vi "RDUW_2.0(old).vi"() -> ()   [LabVIEW 2010]
uses:
  <vilib>/express/express arith-compare/Formula/XNode/ExpressFormulaBlockNode.xnode
panel:
  in  "Current (mA)":dbl
  in  "Laser GPIB":u8=10 max=100
  out "Dummy":string
  out "Dummy angle":i16[](array[numeric])
  out "Quadrant":u8
  out "move y":i32
  out "move x":i32
  out "b":dbl
  out "a":dbl
  out "Arc":dbl
  out "radius":dbl
  in  "Angle":i16
  in  "Y0":i16
  in  "X0":i16
  in  "stop":bool
  out "Loop count":i32
  out "y":i32
  out "x":i32
  out "XY Graph 2":cluster{"Y":dbl[], "Y":dbl[]}[](graph)
  out "x-disp":i32[](array[numeric])
  out "y-disp":i32[](array[numeric])
  in  "Motor GPIB":u8=6
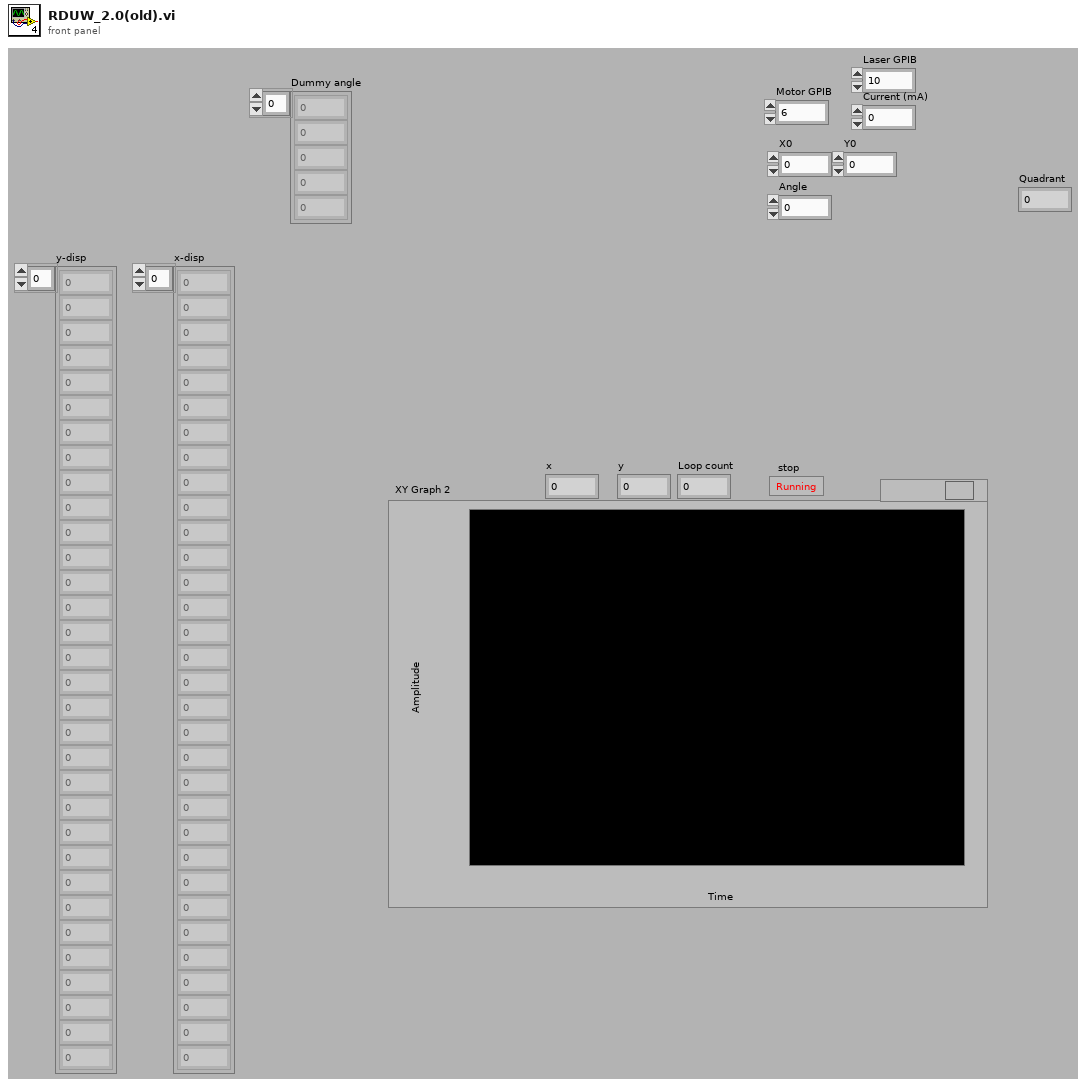
[diagram p1: front panel]
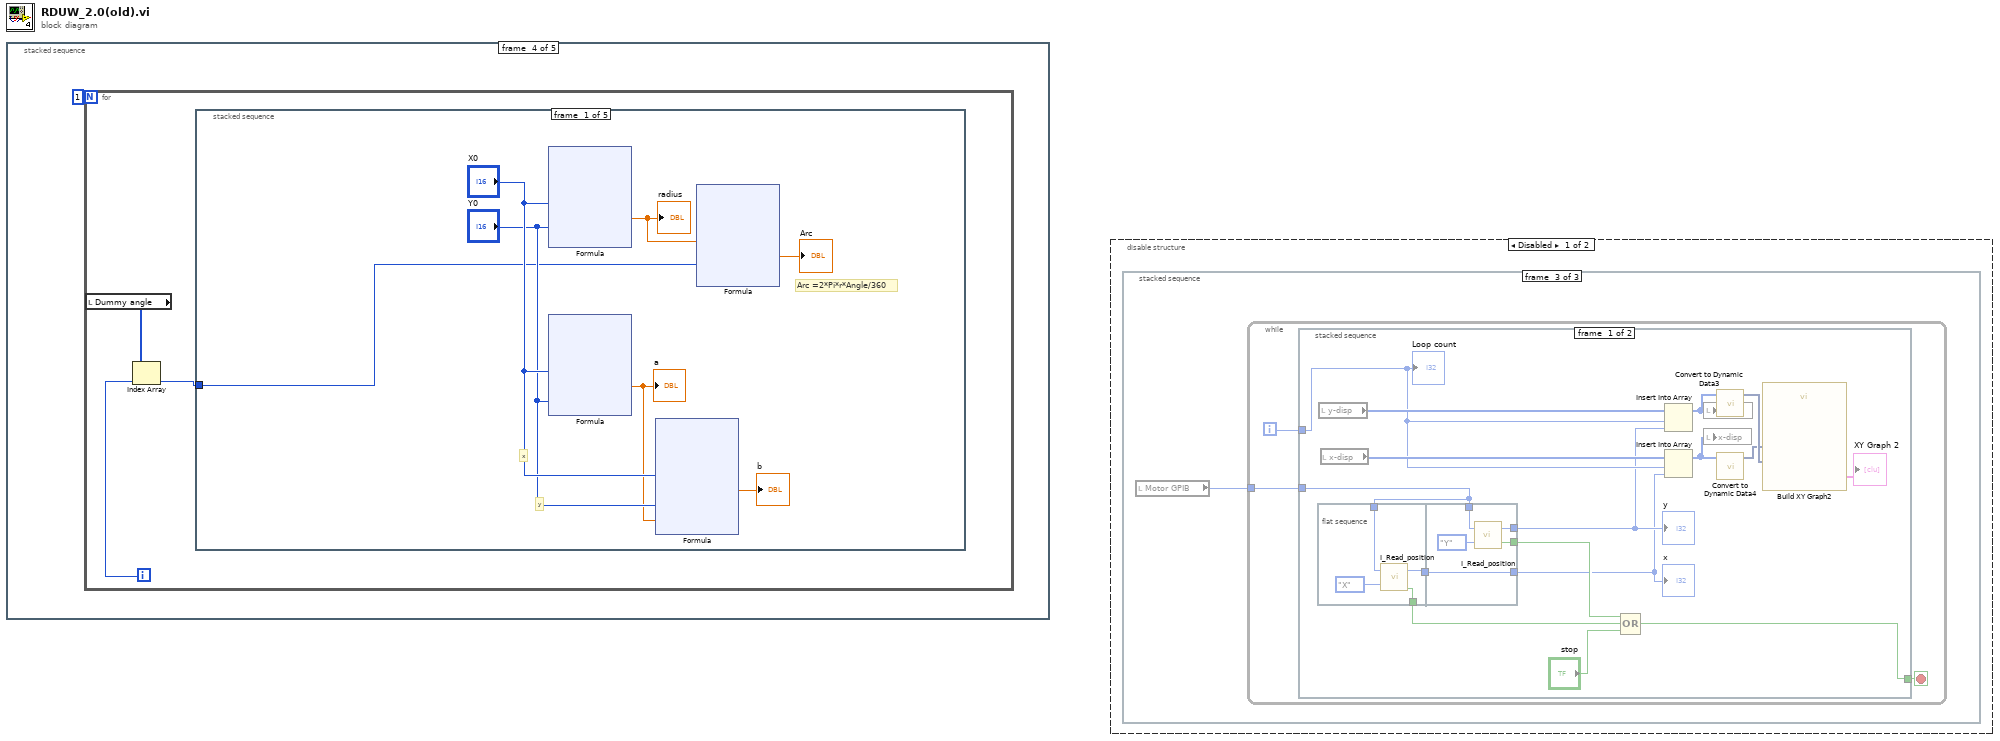
[diagram p0: block diagram]
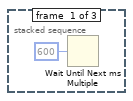
[diagram p2: hidden frame]
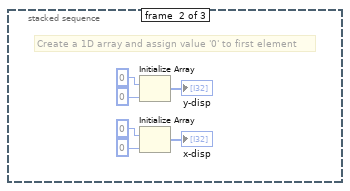
[diagram p3: hidden frame]
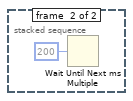
[diagram p4: hidden frame]
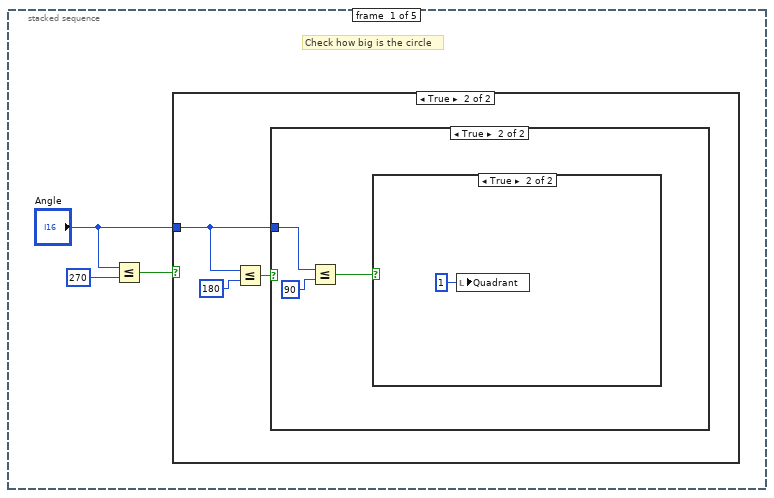
[diagram p6: hidden frame]
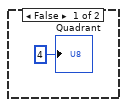
[diagram p7: hidden frame]
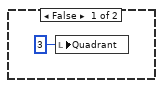
[diagram p8: hidden frame]
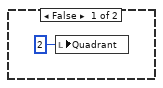
[diagram p9: hidden frame]
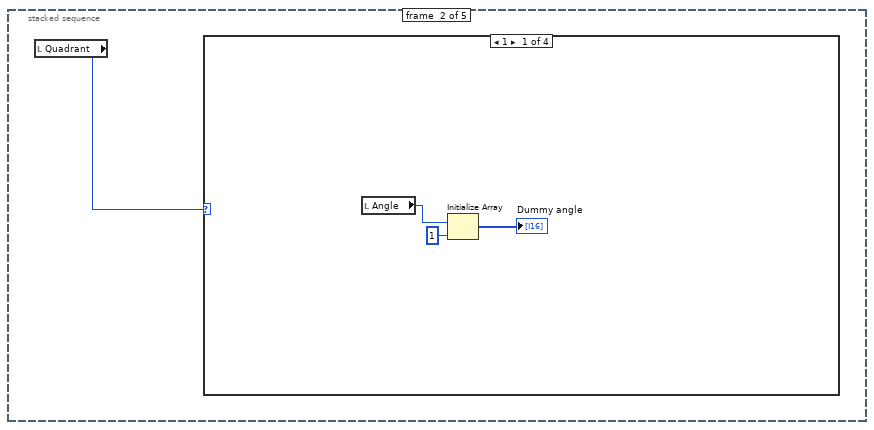
[diagram p10: hidden frame]
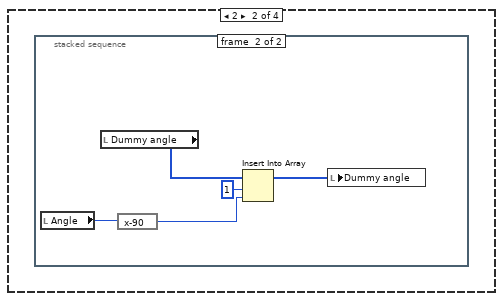
[diagram p11: hidden frame]
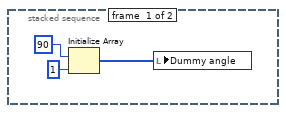
[diagram p12: hidden frame]
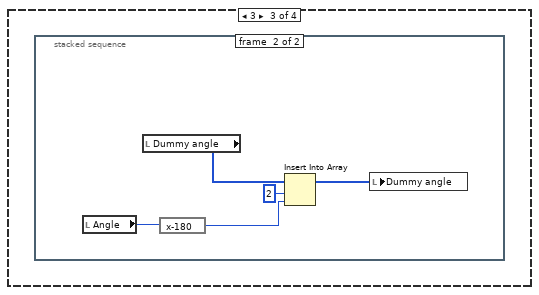
[diagram p13: hidden frame]
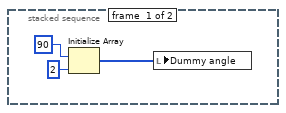
[diagram p14: hidden frame]
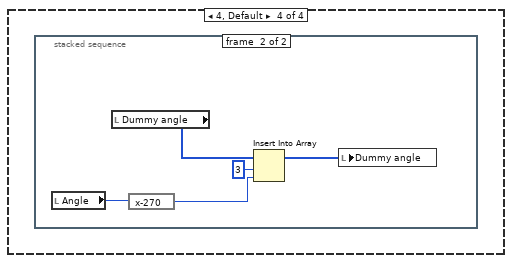
[diagram p15: hidden frame]
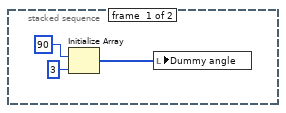
[diagram p16: hidden frame]
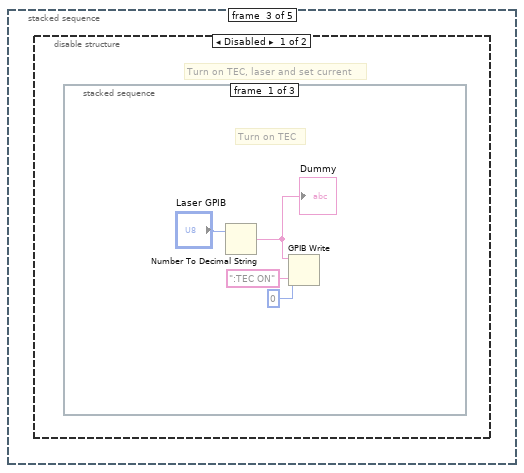
[diagram p17: hidden frame]
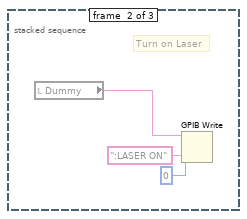
[diagram p18: hidden frame]
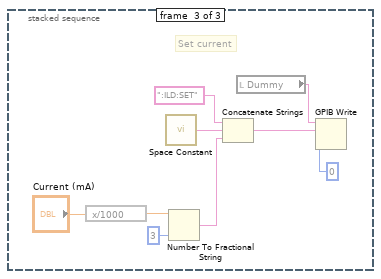
[diagram p19: hidden frame]
diagram:
  n1 = stacked-sequence {
    frame #0 {
      # "Check how big is the circle"
      n2 = Less Or Equal?(x="Angle", y=i16 270) -> (x <= y?=w2:bool)
      n3 = case shown="True" w2 {
        tunnel: "Angle" -> [_ w5]
        frame False {
          "Quadrant" <- u8 4 ("Numeric")
        }
        frame True {
          n4 = Less Or Equal?(x=w5, y=i16 180) -> (x <= y?=w6:bool)
          n5 = case shown="True" w6 {
            tunnel: w5 -> [_ w11]
            frame False {
              n6 = local write "Quadrant"(u8 3 ("Quadrant")) -> ()
            }
            frame True {
              n7 = Less Or Equal?(x=w11, y=i16 90) -> (x <= y?=w9:bool)
              n8 = case shown="True" w9 {
                frame False {
                  n9 = local write "Quadrant"(u8 2 ("Quadrant")) -> ()
                }
                frame True {
                  n10 = local write "Quadrant"(u8 1 ("Quadrant")) -> ()
                }
              }
            }
          }
        }
      }
    }
    frame #1 {
      n11 = local read "Quadrant"() -> (w14:u8)
      n12 = case shown="1" w14 {
        frame 1 {
          n13 = local read "Angle"() -> (w16:i16)
          n14 = Initialize Array(w16, 1 ("dimension size")) -> (→"Dummy angle":i16[])
        }
        frame 2 {
          n15 = stacked-sequence {
            frame #0 {
              n16 = Initialize Array(i16 90 ("element"), 1 ("dimension size")) -> (w20:i16[])
              n17 = local write "Dummy angle"(w20) -> ()
            }
            frame #1 {
              n18 = local read "Angle"() -> (w22:i16)
              n19 = local read "Dummy angle"() -> (w23:i16[])
              n20 = expression code="x-90"(w22) -> (w21:i16)
              n21 = Insert Into Array(array=w23, index=1, new element=w21) -> (w24:i16[])
              n22 = local write "Dummy angle"(w24) -> ()
            }
          }
        }
        frame 3 {
          n23 = stacked-sequence {
            frame #0 {
              n24 = Initialize Array(i16 90 ("element"), 2 ("dimension size")) -> (w28:i16[])
              n25 = local write "Dummy angle"(w28) -> ()
            }
            frame #1 {
              n26 = local read "Angle"() -> (w30:i16)
              n27 = local read "Dummy angle"() -> (w31:i16[])
              n28 = expression code="x-180"(w30) -> (w29:i16)
              n29 = Insert Into Array(array=w31, index=2, new element=w29) -> (w32:i16[])
              n30 = local write "Dummy angle"(w32) -> ()
            }
          }
        }
        frame 4, Default {
          n31 = stacked-sequence {
            frame #0 {
              n32 = Initialize Array(i16 90 ("element"), 3 ("dimension size")) -> (w36:i16[])
              n33 = local write "Dummy angle"(w36) -> ()
            }
            frame #1 {
              n34 = local read "Angle"() -> (w38:i16)
              n35 = local read "Dummy angle"() -> (w39:i16[])
              n36 = expression code="x-270"(w38) -> (w37:i16)
              n37 = Insert Into Array(array=w39, index=3, new element=w37) -> (w40:i16[])
              n38 = local write "Dummy angle"(w40) -> ()
            }
          }
        }
      }
    }
    frame #2 {
      n39 = disable-structure shown="Disabled" {
        frame Disabled {
          # "Turn on TEC, laser and set current"
          n40 = stacked-sequence {
            frame #0 {
              # "Turn on TEC"
              n41 = Number To Decimal String(number="Laser GPIB") -> (decimal integer string=w42:string)  [unwired: 1 in]
              "Dummy" <- w42
              n42 = GPIB Write(0:w42, 1:":TEC ON" ("data"), 2:i16 0 ("mode (0)")) -> ()  [unwired: 2 in, 2 out]
            }
            frame #1 {
              # "Turn on Laser"
              n43 = local read "Dummy"() -> (w46:string)
              n44 = GPIB Write(0:w46, 1:":LASER ON" ("data"), 2:i16 0 ("mode (0)")) -> ()  [unwired: 2 in, 2 out]
            }
            frame #2 {
              # "Set current"
              n45 = expression code="x/1000"("Current (mA)") -> (w53:dbl)
              n46 = call <vilib>:"Space Constant.vi"() -> ("String"=w55:string)
              n47 = Number To Fractional String(number=w53, precision (6)=i16 3) -> (F-format string=w50:string)  [unwired: 2 in]
              n48 = Concatenate Strings(":ILD:SET", w55, w50) -> (w54:string)
              n49 = local read "Dummy"() -> (w49:string)
              n50 = GPIB Write(0:w49, 1:w54, 2:i16 0 ("mode (0)")) -> ()  [unwired: 2 in, 2 out]
            }
          }
        }
        frame Enabled {
        }
      }
    }
    frame #3 {
      n51 = for {
        N: 1 -> [_]
        i -> [w60]
        n52 = local read "Dummy angle"() -> (w61:i16[])
        n53 = Index Array(array=w61, index=w60) -> (element=w59:i16)
        n54 = stacked-sequence {
          tunnel: w59 -> [w62 _ _ w171 _]
          frame #0 {
            # "y"
            # "x"
            # "Arc =2*Pi*r*Angle/360"
            n55 = xnode "Formula"("X1"="X0", "X2"="Y0") -> ("Result"=w68:dbl)  [unwired: 1 in, 1 out]
            "radius" <- w68
            n56 = xnode "Formula"("X1"="X0", "X2"="Y0") -> ("Result"=w64:dbl)  [unwired: 1 in, 1 out]
            "a" <- w64
            n57 = xnode "Formula"("X1"="X0", "X2"="Y0", "X3"=w64) -> ("Result"=→"b":dbl)  [unwired: 1 in, 1 out]
            n58 = xnode "Formula"("X1"=w68, "X2"=w62) -> ("Result"=→"Arc":dbl)  [unwired: 1 in, 1 out]
          }
          frame #1 {
            n59 = local read "radius"() -> (w118:dbl)
            n60 = local read "Angle"() -> (w117:i16)
            n61 = local read "X0"() -> (w113:i16)
            n62 = local read "Y0"() -> (w111:i16)
            n63 = local read "b"() -> (w112:dbl)
            n64 = local read "a"() -> (w114:dbl)
            n65 = xnode "Formula"("r"=w118, "Angle"=w117, "a"=w114, "X0"=w113) -> ("Result"=→"move x":dbl)  [unwired: 2 in, 1 out]
            n66 = xnode "Formula"("a"=w114, "b"=w112, "r"=w118, "Angle"=w117, "X0"=w113, "Y0"=w111) -> ("Result"=→"move y":dbl)  [unwired: 1 in, 1 out]
          }
          frame #2 {
            w153 = u16 10 ("L Speed")
            w163 = u16 10 ("L Speed")
            # "Move Y"
            # "Move X"
            n67 = local read "move x"() -> (w162:i32)
            n68 = Greater?(x=w162, y=0) -> (0:w166:bool)
            n69 = Absolute Value(x=w162) -> (abs(x)=w165:i32)
            n70 = To Unsigned Long Integer(number=w165) -> (unsigned 32bit integer=w164:u32)
            n71 = call "Increment.vi"("GPIB_Addr"="Motor GPIB", "F Speed"=w163, "L Speed"=w163, "Rate"=u16 1, "CCW 3"=w166, "Distance"=w164, "Axis"=enum16{"X", "Y", "Z", "U", "V", "W"}."X") -> ()
            n72 = local read "move y"() -> (w155:i32)
            n73 = local read "Motor GPIB"() -> (w159:u8)
            n74 = Greater?(x=w155, y=0) -> (0:w157:bool)
            n75 = Absolute Value(x=w155) -> (abs(x)=w156:i32)
            n76 = To Unsigned Long Integer(number=w156) -> (unsigned 32bit integer=w154:u32)
            n77 = call "Increment.vi"("GPIB_Addr"=w159, "F Speed"=w153, "L Speed"=w153, "Rate"=u16 1, "CCW 3"=w157, "Distance"=w154, "Axis"=enum16{"X", "Y", "Z", "U", "V", "W"}."Y") -> ()
          }
          frame #3 {
            n78 = local read "Arc"() -> (w174:dbl)
            n79 = expression code="x/19"(w174) -> (w172:dbl)
            n80 = To Long Integer(number=w172) -> (32bit integer=w173:i32)
            n81 = local read "Motor GPIB"() -> (w176:u8)
            n82 = Number To Decimal String(number=w176) -> (decimal integer string=w175:string)  [unwired: 1 in]
            n83 = for {
              N: w173 -> [_]
              tunnel: w175 -> [w182]
              tunnel: w174 -> [w178]
              tunnel: w171 -> [w177]
              i -> [w185]
              # "200*sin[ (i*Pi*200um/s * 95ms)\n/ (180*Arc) ]"
              # "200*cos[ (i*Pi*200um/s * 95ms)\n/ (180*Arc) ]"
              # "y"
              # "x"
              n84 = xnode "Formula"("X1"=w185, "X2"=w177, "X3"=w178) -> ("Result"=w183:dbl)  [unwired: 1 in, 1 out]
              n85 = xnode "Formula"("X1"=w185, "X2"=w177, "X3"=w178) -> ("Result"=w184:dbl)  [unwired: 1 in, 1 out]
              n86 = Wait Until Next ms Multiple(millisecond multiple=u32 95) -> ()  [unwired: 1 out]
              n87 = To Word Integer(number=w184) -> (16bit integer=w187:i16)
              n88 = To Word Integer(number=w183) -> (16bit integer=w194:i16)
              n89 = Number To Decimal String(number=w187) -> (decimal integer string=w186:string)  [unwired: 1 in]
              n90 = Number To Decimal String(number=w194) -> (decimal integer string=w188:string)  [unwired: 1 in]
              n91 = Format Into String(format string="AXI2:SELSP 1:F1 %s:L1 %s:R1 1", w186, w186) -> (resulting string=w189:string)  [unwired: 2 in, 1 out]
              n92 = Format Into String(format string="AXI1:SELSP 2:F2 %s:L2 %s:R2 1", w188, w188) -> (resulting string=w181:string)  [unwired: 2 in, 1 out]
              n93 = call "D200_GPIB.vi"("GPIB\nAddress"=w182, "Write"=TRUE, "Read"=FALSE, "Characters to Write"=w189) -> ()  [unwired: 1 in, 3 out]
              n94 = call "D200_GPIB.vi"("GPIB\nAddress"=w182, "Write"=TRUE, "Read"=FALSE, "Characters to Write"=w181) -> ()  [unwired: 1 in, 3 out]
            }
          }
          frame #4 {
            n95 = disable-structure shown="Disabled" {
              frame Disabled {
                n96 = local read "move x"() -> (w220:i32)
                n97 = local read "move x"() -> (w221:i32)
                n98 = local write "X0"(w221) -> ()
                n99 = local write "Y0"(w220) -> ()
              }
              frame Enabled {
              }
            }
          }
        }
      }
    }
    frame #4 {
      # "Set current to zero after finish drawing the LINE"
      n100 = call <vilib>:"Space Constant.vi"() -> ("String"=w224:string)
      n101 = local read "Dummy"() -> (w227:string)
      n102 = Concatenate Strings(":ILD:SET", w224, "0" ("string")) -> (w225:string)
      n103 = GPIB Write(0:w227, 1:w225, 2:i16 0 ("mode (0)")) -> ()  [unwired: 2 in, 2 out]
    }
  }
  n104 = disable-structure shown="Disabled" {
    frame Disabled {
      n105 = stacked-sequence {
        frame #0 {
          n106 = Wait Until Next ms Multiple(millisecond multiple=u32 600) -> ()  [unwired: 1 out]
        }
        frame #1 {
          # "Create a 1D array and assign value '0' to first element"
          n107 = Initialize Array(0 ("element"), 0 ("dimension size")) -> (→"y-disp":i32[])
          n108 = Initialize Array(0 ("element"), 0 ("element")) -> (→"x-disp":i32[])
        }
        frame #2 {
          n109 = local read "Motor GPIB"() -> (w235:u8)
          n110 = while {
            tunnel: w235 -> [w236]
            i -> [w238]
            stop <- w237 stop-if-true
            n111 = stacked-sequence {
              tunnel: w238 -> [w248 _]
              tunnel: [w245 _] -> w237
              tunnel: w236 -> [w244 _]
              frame #0 {
                n112 = flat-sequence {
                  tunnel: [w258] -> w247
                  tunnel: w244 -> [w257]
                  tunnel: [w255] -> w254
                  tunnel: w244 -> [w263]
                  tunnel: [w262] -> w243
                  tunnel: [w261] -> w242
                  tunnel: w254 -> [w259]
                  tunnel: [w259] -> w241
                  frame #0 {
                    n113 = call "I_Read_position.vi"("Axis"=enum16{"X", "Y", "Z"}."X", "Motor GPIB"=w257) -> ("Error?"=w258:bool, "Position"=w255:i32)
                  }
                  frame #1 {
                    n114 = call "I_Read_position.vi"("Axis"=enum16{"X", "Y", "Z"}."Y", "Motor GPIB"=w263) -> ("Error?"=w261:bool, "Position"=w262:i32)
                  }
                }
                n115 = local read "y-disp"() -> (w252:i32[])
                n116 = local read "x-disp"() -> (w253:i32[])
                n117 = Compound Arithmetic op=OR(w242, w247, "stop") -> (w245:bool)
                n118 = Insert Into Array(array=w252, index=w248, new element=w243) -> (w251:i32[])
                n119 = Insert Into Array(array=w253, index=w248, new element=w241) -> (w250:i32[])
                n120 = local write "y-disp"(w251) -> ()
                n121 = local write "x-disp"(w250) -> ()
                n122 = call "Convert to Dynamic Data3"("Array"=w251) -> ("Dynamic Data Type"=w240:dynamicdata)  [unwired: 3 in]
                n123 = call "Convert to Dynamic Data4"("Array"=w250) -> ("Dynamic Data Type"=w239:dynamicdata)  [unwired: 3 in]
                n124 = call "Build XY Graph2"("Y Input"=w240, "X Input"=w239) -> ("XY Graph"=→"XY Graph 2":cluster{"Y":dbl[], "Y":dbl[]}[])  [unwired: 3 in, 6 out]
                "Loop count" <- w248
                "y" <- w243
                "x" <- w241
              }
              frame #1 {
                n125 = Wait Until Next ms Multiple(millisecond multiple=u32 200) -> ()  [unwired: 1 out]
              }
            }
          }
        }
      }
    }
    frame Enabled {
    }
  }
